vi "Get State.vi"(1 "Hash Function in":refnum<class "NI_SHA-3.lvclass">) -> (0 "state array":T1 {"A24" format="%016x"; "A23" format="%016x"; "A22" format="%016x"; "A21" format="%016x"; "A20" format="%016x"; "A19" format="%016x"; "A18" format="%016x"; "A17" format="%016x"; "A16" format="%016x"; "A15" format="%016x"; "A14" format="%016x"; "A13" format="%016x"; "A12" format="%016x"; "A11" format="%016x"; "A10" format="%016x"; "A09" format="%016x"; "A08" format="%016x"; "A07" format="%016x"; "A06" format="%016x"; "A05" format="%016x"; "A04" format="%016x"; "A03" format="%016x"; "A02" format="%016x"; "A01" format="%016x"; "A00" format="%016x"})   [LabVIEW 2020, in "NI_SHA-3.lvclass"]
uses:
  <vilib>/security/Message Digest/SHA-3/NI_SHA-3.lvclass
  <vilib>/security/Message Digest/SHA-3/subVIs/state.ctl
  <vilib>/security/Message Digest/SHA-3/subVIs/state word.ctl
  <vilib>/security/Message Digest/SHA-3/NI_SHA-3.lvclass/NI_SHA-3.ctl
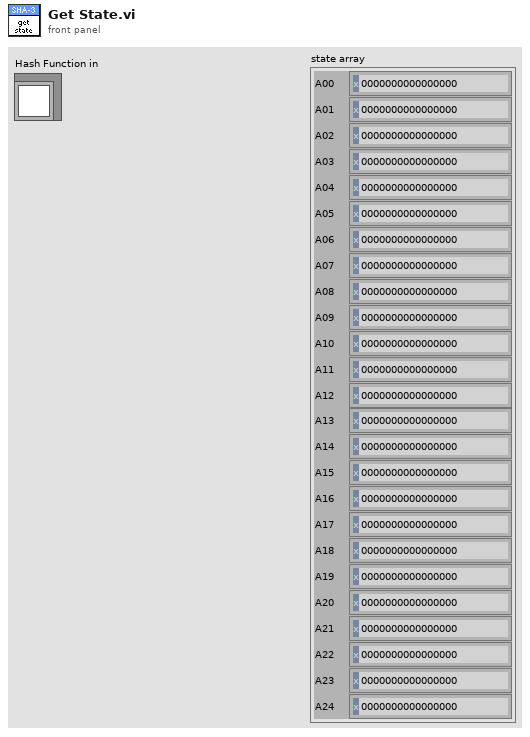
[diagram p1: front panel]
types:
  T1 = typedef "NI_SHA-3.lvclass/state.ctl" = cluster{"A00":T2, "A01":T2, "A02":T2, "A03":T2, "A04":T2, "A05":T2, "A06":T2, "A07":T2, "A08":T2, "A09":T2, "A10":T2, "A11":T2, "A12":T2, "A13":T2, "A14":T2, "A15":T2, "A16":T2, "A17":T2, "A18":T2, "A19":T2, "A20":T2, "A21":T2, "A22":T2, "A23":T2, "A24":T2}
  T2 = typedef "NI_SHA-3.lvclass/state word.ctl" = u64
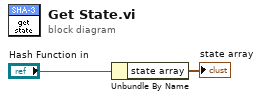
[diagram p0: block diagram]
diagram:
  n1 = Unbundle By Name("Hash Function in") -> ("state array"=→"state array":T1)
